vi "Error Handler FGV.vi"(8 "error in (no error)":errorcluster, 10 "Action":T1=enum."System Error", 11 "Application to EH":refnum<class "Simulation Interface.lvclass">) -> (0 "error out":errorcluster)   [LabVIEW 2012, in "Architecture.lvlib" / "Error Handler.lvclass"]
uses:
  Error Handler.lvclass
  Simulation Interface/Simulation Interface.lvclass
  Thread/Thread.lvclass
  Wash Abort State/Wash Abort Terminate State.lvclass
  Queue/Queue.lvclass
  Stop Message/Stop Msg.lvclass
  Car Wash Controller/Car Wash Controller.lvclass
  Entry Console/Entry Console.lvclass
  Vehicle Position Simulation/Vehicle Position Simulation.lvclass
  Wash Display Console/Wash Display Console.lvclass
  EH Action.ctl
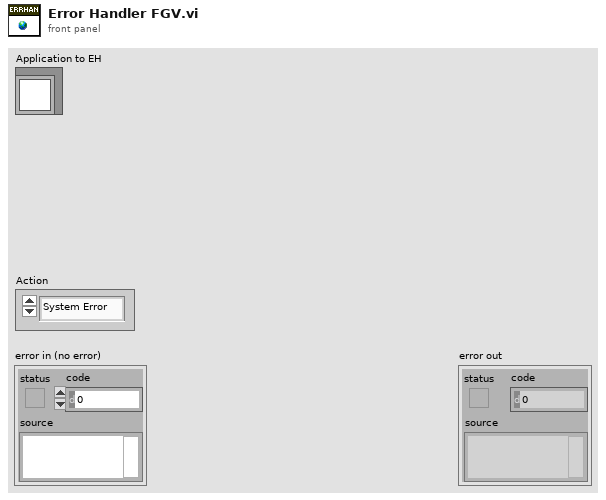
[diagram p1: front panel]
types:
  T1 = typedef "Architecture.lvlib/Error Handler.lvclass/EH Action.ctl" = enum16{"Define Threads", "Close", "System Error", "Wash Cycle Error", "Minor Error", "Initialize"}
  T2 = enum16{"open", "replace", "create", "open or create", "replace or create", "replace or create with confirmation"}
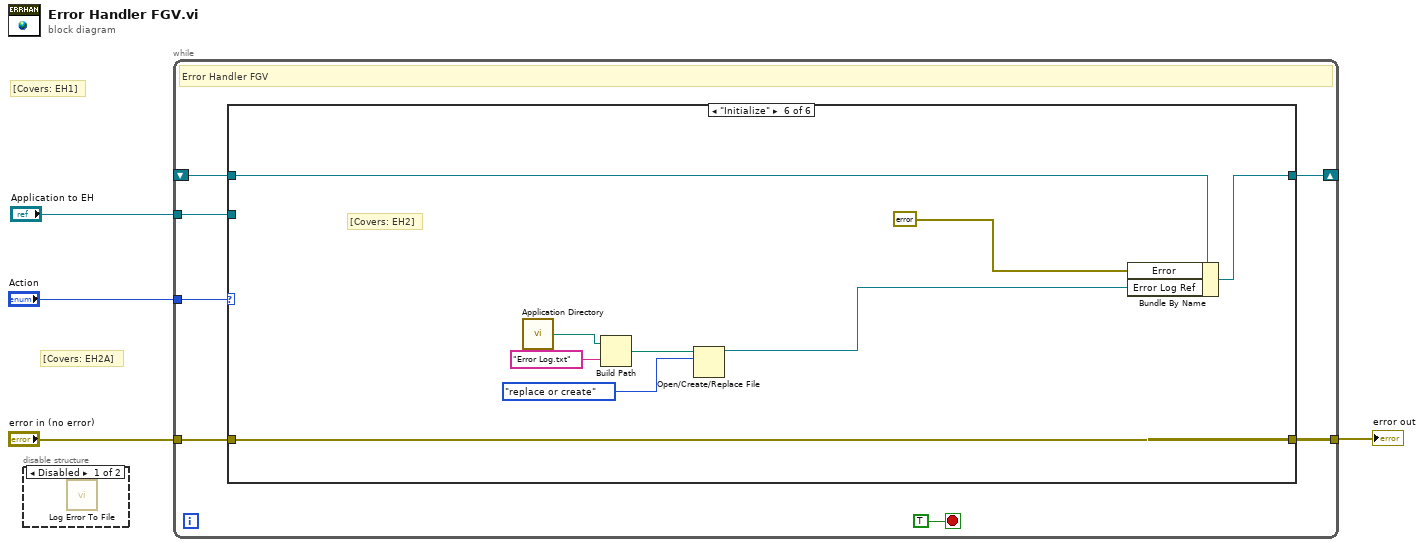
[diagram p0: block diagram]
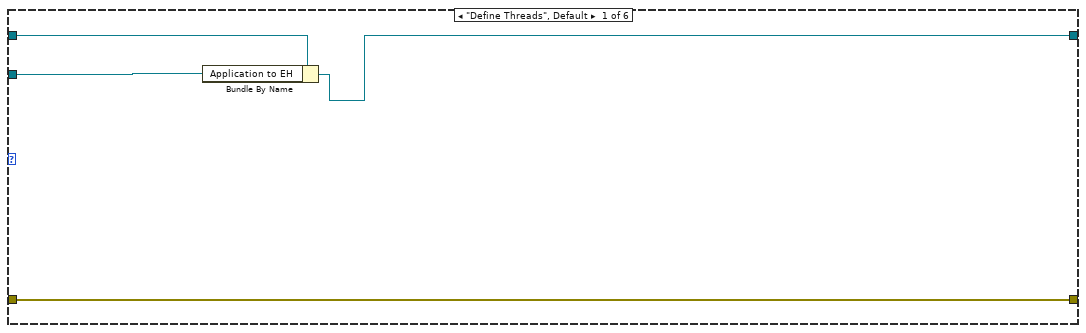
[diagram p3: hidden frame]
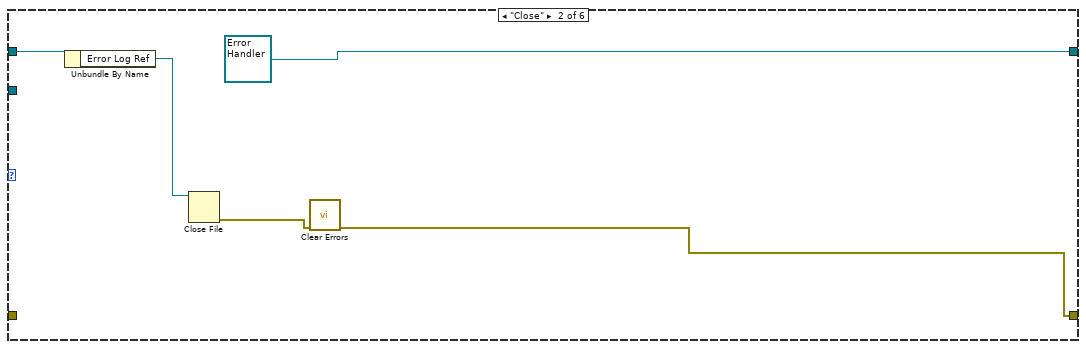
[diagram p4: hidden frame]
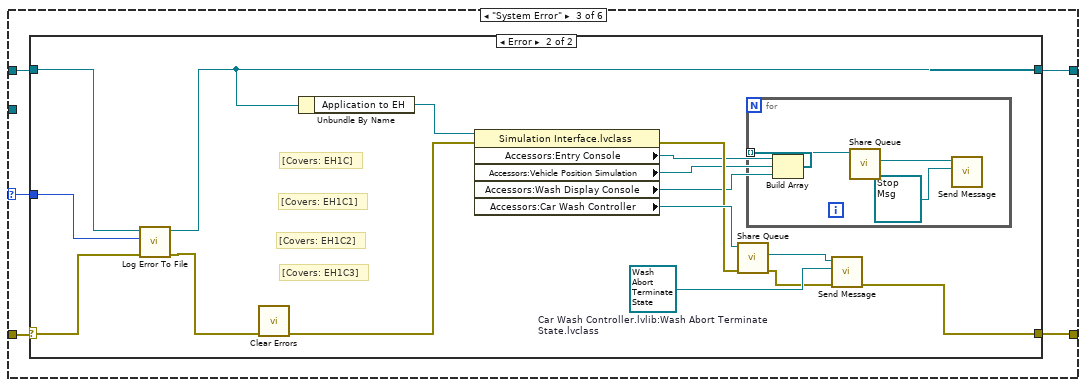
[diagram p5: hidden frame]
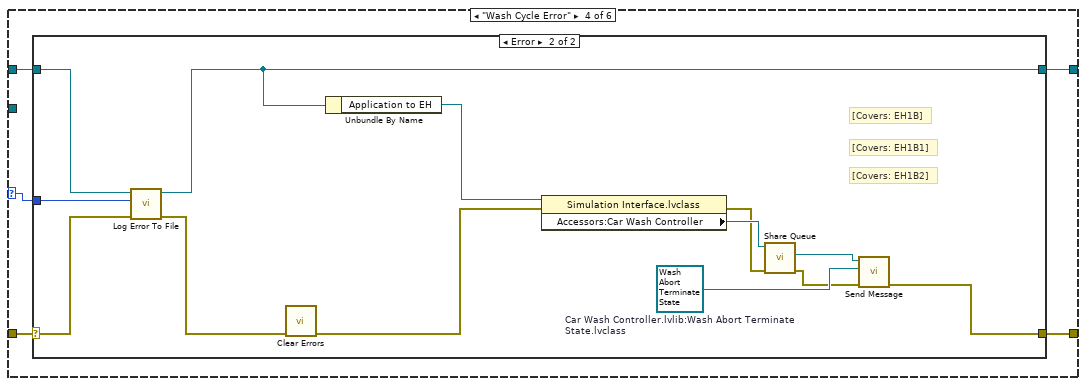
[diagram p7: hidden frame]
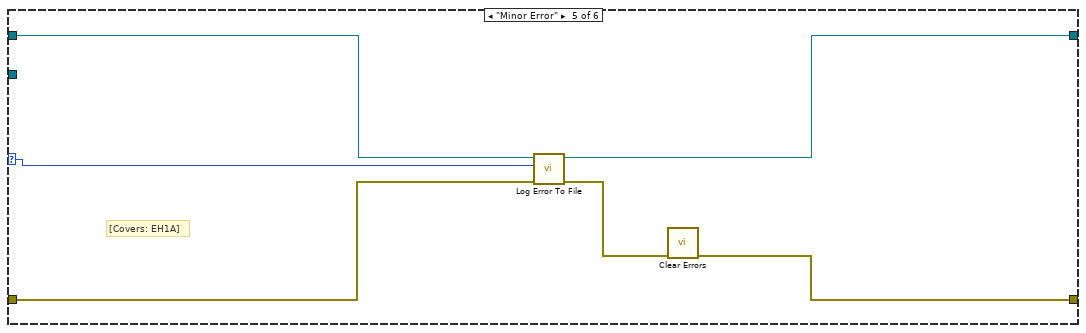
[diagram p9: hidden frame]
diagram:
  # "[Covers: EH2A]"
  # "[Covers: EH1]"
  n1 = disable-structure shown="Disabled" {
    frame Disabled {
      n2 = call "Log Error To File.vi"() -> ()  [unwired: 10 in, 2 out]
    }
    frame Enabled {
    }
  }
  n3 = while {
    shift-right: [w11] -> _
    shift-left: _ -> [w9]
    tunnel: "Action" -> [w10]
    tunnel: [w8] -> w3
    tunnel: "error in (no error)" -> [w7]
    tunnel: "Application to EH" -> [w6]
    stop <- TRUE stop-if-true
    # "Error Handler FGV"
    n4 = case shown="\"Initialize\"" w10 {
      selector: w10 -> [_ _ w21 w48 w68 _]
      tunnel: [w13 refnum<class "Error Handler.lvclass"> refnum ("Error Handler in") w22 w50 w72 w81] -> w11
      tunnel: w9 -> [w14 w19 w25 w52 w73 w82]
      tunnel: [w15 w16 w23 w49 w69 w74] -> w8
      tunnel: w7 -> [w15 _ w24 w51 w71 w74]
      tunnel: w6 -> [w12 _ _ _ _ _]
      frame "Define Threads", Default {
        n5 = Bundle By Name(cluster=w14, "Application to EH"=w12) -> (w13:refnum<class "Error Handler.lvclass">)
      }
      frame "Close" {
        n6 = Unbundle By Name(w19) -> ("Error Log Ref"=w18:refnum<file>)
        n7 = Close File(refnum=w18) -> (error out=w17:errorcluster)  [unwired: 1 in, 1 out]
        n8 = call <vilib>:"Clear Errors.vi"("error in (no error)"=w17) -> ("error out"=w16:errorcluster)  [unwired: 5 in, 1 out]
      }
      frame "System Error" {
        n9 = case shown="Error" w24 {
          selector: w24 -> [w26 w32]
          tunnel: w25 -> [w27 w30]
          tunnel: [w27 w29] -> w22
          tunnel: [w26 w37] -> w23
          tunnel: w21 -> [_ w28]
          frame No Error {
          }
          frame Error {
            w40 = refnum<class "Wash Abort Terminate State.lvclass"> refnum  # Car Wash Controller.lvlib:Wash Abort Terminate State.lvclass
            # "[Covers: EH1C3]"
            # "[Covers: EH1C2]"
            # "[Covers: EH1C1]"
            # "[Covers: EH1C]"
            n10 = call "Log Error To File.vi"("Error In"=w32, "Error Level"=w28, "Error Handler in"=w30) -> ("error out"=w31:errorcluster, "Error Handler out"=w29:refnum<class "Error Handler.lvclass">)  [unwired: 7 in]
            n11 = call <vilib>:"Clear Errors.vi"("error in (no error)"=w31) -> ("error out"=w42:errorcluster)  [unwired: 5 in, 1 out]
            n12 = Unbundle By Name(w29) -> ("Application to EH"=w44:refnum<class "Simulation Interface.lvclass">)
            n13 = property class="Simulation Interface.lvclass"(reference=w44, error in=w42) -> (error out=w39:errorcluster, "Accessors:Entry Console"=w36:refnum<class "Entry Console.lvclass">, "Accessors:Vehicle Position Simulation"=w35:refnum<class "Vehicle Position Simulation.lvclass">, "Accessors:Wash Display Console"=w34:refnum<class "Wash Display Console.lvclass">, "Accessors:Car Wash Controller"=w43:refnum<class "Car Wash Controller.lvclass">)  [unwired: 1 out]
            n14 = call "Share Queue.vi"("error in (no error)"=w39, "Thread in"=w43) -> ("error out"=w38:errorcluster, "Architecture.lvlib:Queue.lvclass"=w41:refnum<class "Queue.lvclass">)  [unwired: 7 in, 1 out]
            n15 = Build Array(w36, w35, w34) -> (w33:refnum<class "Thread.lvclass">[])
            n16 = for {
              tunnel: w33 -> [w47] mode=indexing
              n17 = call "Share Queue.vi"("Thread in"=w47) -> ("Architecture.lvlib:Queue.lvclass"=w46:refnum<class "Queue.lvclass">)  [unwired: 8 in, 2 out]
              n18 = call "Send Message.vi"("Architecture.lvlib:Message.lvclass"=refnum<class "Stop Msg.lvclass"> refnum ("Architecture.lvlib:Stop Msg.lvclass"), "Queue in"=w46) -> ()  [unwired: 8 in, 2 out]
            }
            n19 = call "Send Message.vi"("error in (no error)"=w38, "Architecture.lvlib:Message.lvclass"=w40, "Queue in"=w41) -> ("error out"=w37:errorcluster)  [unwired: 7 in, 1 out]
          }
        }
      }
      frame "Wash Cycle Error" {
        n20 = case shown="Error" w51 {
          selector: w51 -> [w53 w59]
          tunnel: w52 -> [w54 w58]
          tunnel: [w54 w57] -> w50
          tunnel: [w53 w60] -> w49
          tunnel: w48 -> [_ w55]
          frame No Error {
          }
          frame Error {
            w63 = refnum<class "Wash Abort Terminate State.lvclass"> refnum  # Car Wash Controller.lvlib:Wash Abort Terminate State.lvclass
            # "[Covers: EH1B2]"
            # "[Covers: EH1B1]"
            # "[Covers: EH1B]"
            n21 = call "Log Error To File.vi"("Error In"=w59, "Error Level"=w55, "Error Handler in"=w58) -> ("error out"=w56:errorcluster, "Error Handler out"=w57:refnum<class "Error Handler.lvclass">)  [unwired: 7 in]
            n22 = call <vilib>:"Clear Errors.vi"("error in (no error)"=w56) -> ("error out"=w65:errorcluster)  [unwired: 5 in, 1 out]
            n23 = Unbundle By Name(w57) -> ("Application to EH"=w67:refnum<class "Simulation Interface.lvclass">)
            n24 = property class="Simulation Interface.lvclass"(reference=w67, error in=w65) -> (error out=w62:errorcluster, "Accessors:Car Wash Controller"=w66:refnum<class "Car Wash Controller.lvclass">)  [unwired: 1 out]
            n25 = call "Share Queue.vi"("error in (no error)"=w62, "Thread in"=w66) -> ("error out"=w61:errorcluster, "Architecture.lvlib:Queue.lvclass"=w64:refnum<class "Queue.lvclass">)  [unwired: 7 in, 1 out]
            n26 = call "Send Message.vi"("error in (no error)"=w61, "Architecture.lvlib:Message.lvclass"=w63, "Queue in"=w64) -> ("error out"=w60:errorcluster)  [unwired: 7 in, 1 out]
          }
        }
      }
      frame "Minor Error" {
        # "[Covers: EH1A]"
        n27 = call "Log Error To File.vi"("Error In"=w71, "Error Level"=w68, "Error Handler in"=w73) -> ("error out"=w70:errorcluster, "Error Handler out"=w72:refnum<class "Error Handler.lvclass">)  [unwired: 7 in]
        n28 = call <vilib>:"Clear Errors.vi"("error in (no error)"=w70) -> ("error out"=w69:errorcluster)  [unwired: 5 in, 1 out]
      }
      frame "Initialize" {
        # "[Covers: EH2]"
        n29 = call <vilib>:"Application Directory.vi"() -> ("Application Directory"=w79:path)
        n30 = Build Path(base path=w79, name or relative path="Error Log.txt") -> (appended path=w77:path)
        n31 = Open/Create/Replace File(file path (use dialog)=w77, operation (0:open)=T2."replace or create") -> (refnum out=w75:refnum<file>)  [unwired: 4 in, 2 out]
        n32 = Bundle By Name(cluster=w82, "Error"=errorcluster {"status"=FALSE, "code"=0, "source"=""}, "Error Log Ref"=w75) -> (w81:refnum<class "Error Handler.lvclass">)
      }
    }
  }
  "error out" <- w3
